vi "REF.vi"(0 "System no.":i32=1 min=1 max=4 step=1, 2 "Affected axes":string[](array[string]), 3 "All axes?":bool, 5 "error in":errorcluster, 12 "Stop refnum":refnum<vi>) -> (14 "REF successful?":bool[](array[boolean]), 19 "error out":errorcluster)   [LabVIEW 2026]
doc: "Moves the specified axes to the reference position, waits until this position is reached (polling with #7), and indicates whether referencing was successful or not. VI will also stop if Stop refnum or Local stop is TRUE.\n\nC-880K005: VI only supported when called through PI_Multix.vi"
panel:
  in  "Local stop":bool
  # "Moves the specified axes to the reference position, waits\nuntil this position is reached (polling with #7) and indicates\nwhether referencing was successful or not. VI will also stop\nif Stop refnum or Local stop is TRUE."
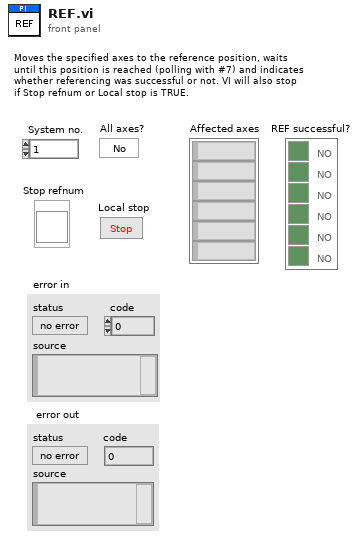
[diagram p1: front panel]
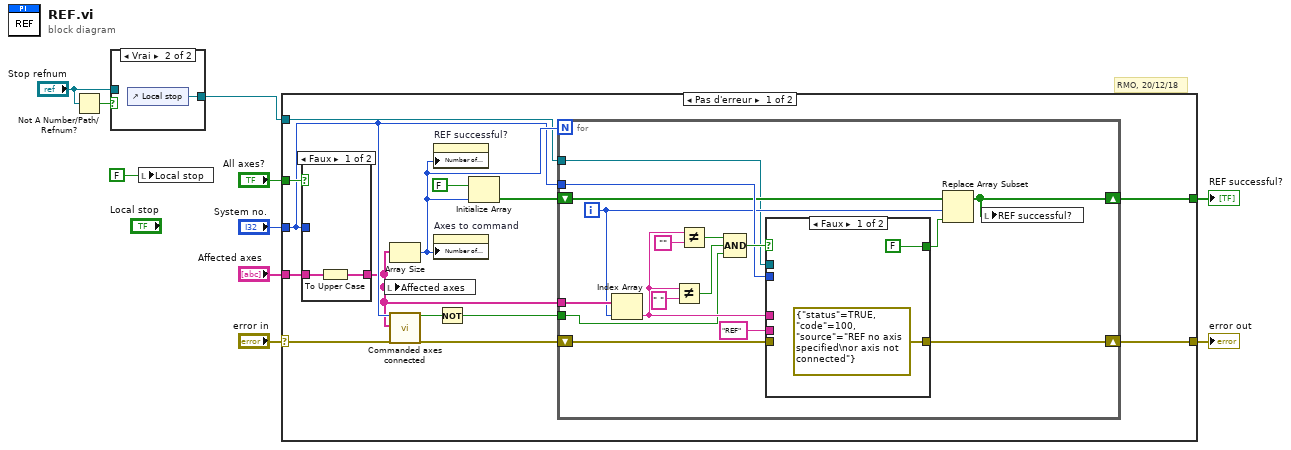
[diagram p0: block diagram]
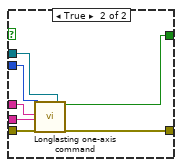
[diagram p3: hidden frame]
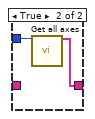
[diagram p4: hidden frame]
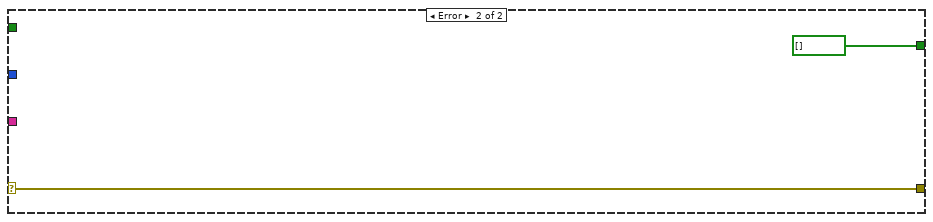
[diagram p5: hidden frame]
diagram:
  # "RMO, 20/12/18"
  n1 = Not A Number/Path/Refnum?(number/path/refnum="Stop refnum") -> (NaN/Path/Refnum?=w6:bool)
  n2 = case shown="Vrai" w6 {
    tunnel: [w11 w12] -> w4
    tunnel: "Stop refnum" -> [w11 _]
    frame False {
    }
    frame True {
      n3 = control-ref of="Local stop"() -> (w12:refnum<vi>)
    }
  }
  n4 = local write "Local stop"(FALSE ("Local stop")) -> ()
  n5 = case shown="Pas d'erreur" "error in" {
    selector: "error in" -> [w15 w58]
    tunnel: "All axes?" -> [w26 _]
    tunnel: "System no." -> [w22 _]
    tunnel: [w16 w58] -> w8
    tunnel: w4 -> [w17 _]
    tunnel: [w14 bool[] []] -> w2
    tunnel: "Affected axes" -> [w13 _]
    frame No Error {
      n6 = case shown="Faux" w26 {
        tunnel: w22 -> [_ w56]
        tunnel: [w54 w55] -> w21
        tunnel: w13 -> [w53 _]
        frame False {
          n7 = To Upper Case(1:w53) -> (0:w54:string[])
        }
        frame True {
          n8 = call "Get all axes.vi"("System no."=w56) -> ("Conn. Axes"=w55:string[])  [unwired: 18 out]
        }
      }
      n9 = local write "Affected axes"(w21) -> ()
      n10 = Array Size(array=w21) -> (size(s)=w25:i32)
      n11 = call "Commanded axes connected.vi"("System no."=w22, "Commanded axes"=w21, "error in"=w15) -> ("Controller error"=w19:bool, "error out"=w20:errorcluster)  [unwired: 15 out]
      n12 = property on="REF successful?" class="Tabl (strict)"("Number of Rows"=w25) -> ()  [unwired: 2 in, 2 out]
      n13 = property on="Axes to command" class="Tabl (strict)"("Number of Rows"=w25) -> ()  [unwired: 2 in, 2 out]
      n14 = Not(x=w19) -> (.not. x?=w18:bool)
      n15 = Initialize Array(FALSE, w25) -> (w23:bool[])
      n16 = for {
        N: w25 -> [_]
        tunnel: w21 -> [w43]
        tunnel: w22 -> [w37]
        shift-right: [w35] -> w16
        shift-left: w20 -> [w34]
        shift-right: [w27] -> w14
        shift-left: w23 -> [w30]
        tunnel: w18 -> [w29]
        tunnel: w17 -> [w28]
        i -> [w32]
        n17 = Index Array(array=w43, index=w32) -> (element=w36:string)
        n18 = Not Equal?(x=w36, y=" ") -> (x != y?=w39:bool)
        n19 = Not Equal?(x=w36, y="") -> (x != y?=w40:bool)
        n20 = Compound Arithmetic op=AND(w40, w39, w29) -> (w38:bool)
        n21 = case shown="Faux" w38 {
          tunnel: w37 -> [_ w52]
          tunnel: w36 -> [_ w51]
          tunnel: [errorcluster {"status"=TRUE, "code"=100, "source"="REF no axis specified\nor axis not connected"} ("error out") w50] -> w35
          tunnel: w34 -> [_ w49]
          tunnel: "REF" -> [_ w48]
          tunnel: [FALSE w47] -> w31
          tunnel: w28 -> [_ w46]
          frame False {
          }
          frame True {
            n22 = call "Longlasting one-axis command.vi"("System no."=w52, "Axis to command"=w51, "Command"=w48, "error in"=w49, "Stop refnum"=w46) -> ("Answer"=w47:bool, "error out"=w50:errorcluster)  [unwired: 2 in, 11 out]
          }
        }
        n23 = Replace Array Subset(array=w30, new element=w31, index=w32) -> (w27:bool[])
        n24 = local write "REF successful?"(w27) -> ()
      }
    }
    frame Error {
    }
  }
  "error out" <- w8
  "REF successful?" <- w2
